vi "Untitled 1.vi"() -> ()   [LabVIEW 2010]
uses:
  Source Code/SubVIs/ModBUS Driver/Private/MBDRV_Action.ctl
  Source Code/SubVIs/ModBUS Driver/Private/MBDRV_Response.ctl
  Source Code/SubVIs/ModBUS Driver/Private/MBDRV_Response List.ctl
  Server/Serial Config.ctl
  Source Code/SubVIs/ModBUS Driver/Private/MBDRV_Command Data.ctl
  Source Code/SubVIs/ModBUS Driver/Private/MBDRV_Command List.ctl
  server.ctl
panel:
  in  "Radio Buttons":enum32{"Boolean", "Boolean 2", "Boolean 3"}(radio)
  in  "Tab Control":T1(tab)
  out "Response List":T2
  in  "Start":bool
  in  "Stop":bool
  in  "Exit":bool
  in  "Config":bool
  in  "Serial Config":T5={"串口选择"="COM1", "通讯速率"=9600, "超时时间"=200, "数据位长"=8, "奇偶校验"=enum."Even", "停止位长"=10, "握手控制"=0, "字符结束"=TRUE, "结束字符"=10, "仪器地址"=1, "刷新时间"=2.0} {"结束字符" format="%.0x"; "握手控制" items=["None", "XON/XOFF", "RTS/CTS", "XON/XOFF & RTS/CTS", "DTR/DSR", "XON/XOFF & DTR/DSR"]; "停止位长" items=["1.0"=10, "1.5"=15, "2.0"=20]; "数据位长" min=5 max=8 step=1}
  in  "Command":bool
  in  "Write To PLC":T6
  out "Read From PLC":T2
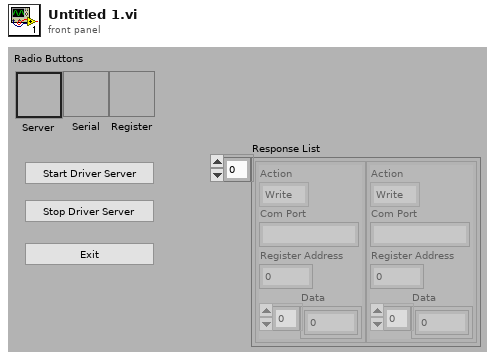
[diagram p1: front panel]
types:
  T1 = enum32{"Server Config", "Serial Config", "Write Registers"}
  T2 = typedef "MBDRV_Response List.ctl" = T3[]
  T3 = typedef "MBDRV_Response.ctl" = cluster{"Action":T4, "Com Port":string, "Register Address":u16, "Data":i16[]}
  T4 = typedef "MBDRV_Action.ctl" = enum16{"Write", "Read"}
  T5 = typedef "Serial Config.ctl" = cluster{"串口选择":refnum<visa-resource-name>, "通讯速率":u32, "超时时间":u32, "数据位长":u16, "奇偶校验":enum16{"None", "Odd", "Even", "Mark", "Space"}, "停止位长":u16, "握手控制":u16, "字符结束":bool, "结束字符":u8, "仪器地址":u32, "刷新时间":dbl}
  T6 = typedef "MBDRV_Command List.ctl" = T7[]
  T7 = typedef "MBDRV_Command Data.ctl" = cluster{"Action":T4, "Com Port":string, "Register Address":u16, "Data To Write/Num To Read":i16}
  T8 = typedef "LVRectTypeDef.ctl" = cluster{"left":i16, "top":i16, "right":i16, "bottom":i16}
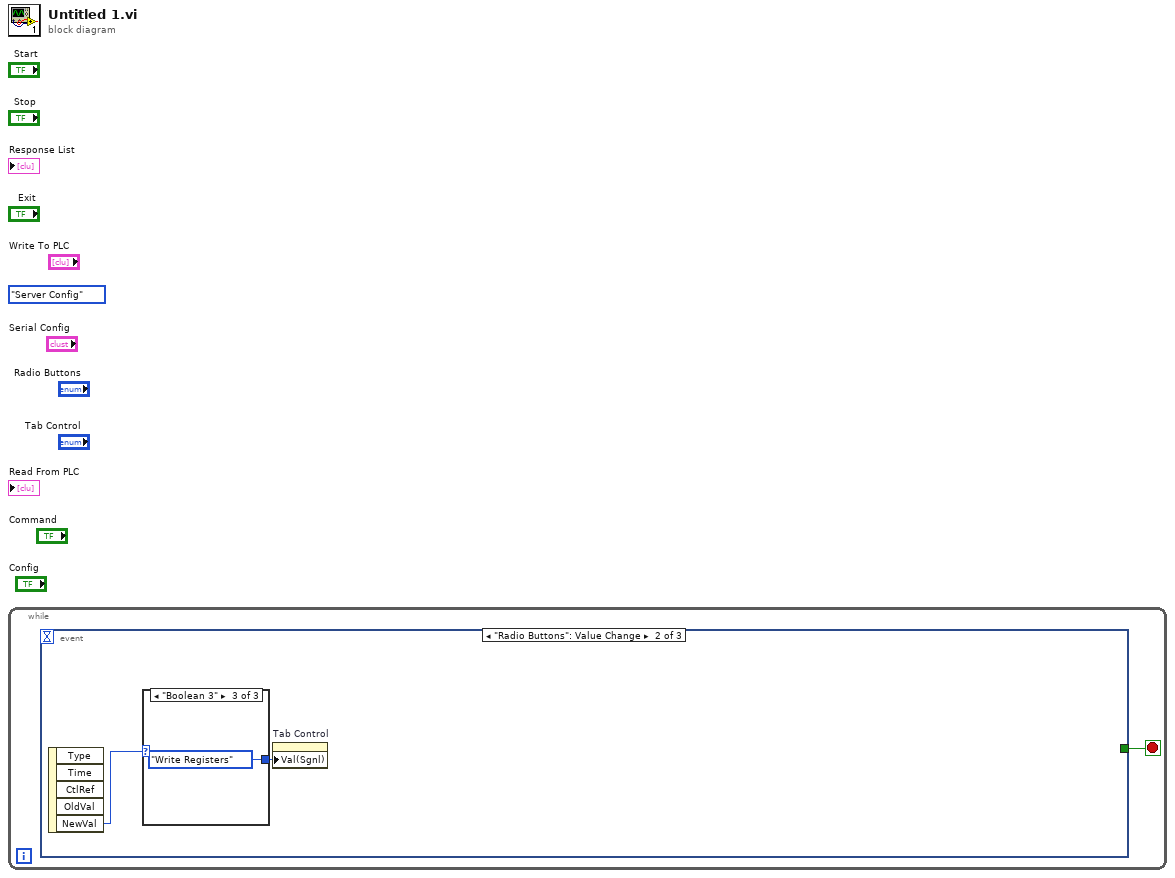
[diagram p0: block diagram]
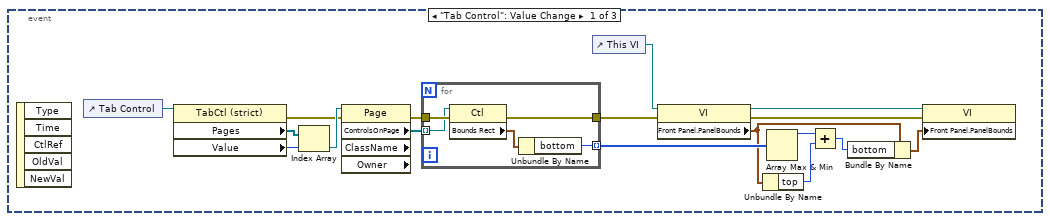
[diagram p2: hidden frame]
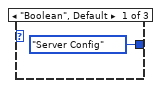
[diagram p3: hidden frame]
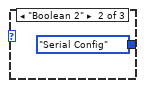
[diagram p4: hidden frame]
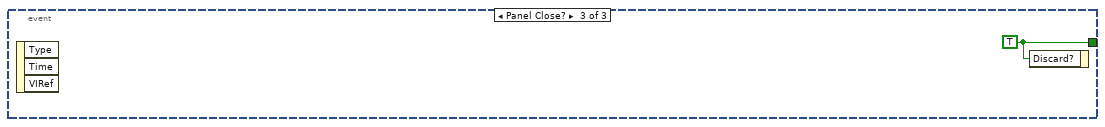
[diagram p5: hidden frame]
diagram:
  (unwired) T1."Server Config" ("Tab Control")
  n1 = while {
    stop <- w1 stop-if-true
    n2 = event shown="[1] \"Radio Buttons\": Value Change" {
      selector: _ -> [_ _ _]
      dyn-events: _ -> [_ _ _]
      timeout: _ -> [_ _ _]
      tunnel: [_ _ w29] -> w1
      event "Tab Control": Value Change {
        n3 = event-data() -> ()  [unwired: 1 in, 5 out]
        n4 = control-ref of="Tab Control"() -> (w4:refnum<vi>)
        n5 = property class="TabCtl (strict)"(reference=w4) -> (error out=w8:errorcluster, "Pages"=w18:refnum<vi>[], "Value"=w17:T1)  [unwired: 1 in, 1 out]
        n6 = Index Array(array=w18, index=w17) -> (element=w15:refnum<vi>)
        n7 = property class="Page" props=["ControlsOnPage", "ClassName", "Owner"](reference=w15, error in=w8) -> (error out=w7:errorcluster, "ControlsOnPage"=w16:refnum<vi>[])  [unwired: 3 out]
        n8 = for {
          tunnel: w16 -> [w19] mode=indexing
          tunnel: [w20] -> w14 mode=indexing
          tunnel: w7 -> [w23]
          tunnel: [w22] -> w6
          n9 = property class="Ctl"(reference=w19, error in=w23) -> (error out=w22:errorcluster, "Bounds Rect"=w21:T8)  [unwired: 1 out]
          n10 = Unbundle By Name(w21) -> ("bottom"=w20:i16)
        }
        n11 = control-ref of="This VI"() -> (w13:refnum<vi>)
        n12 = property class="VI"(reference=w13, error in=w6) -> (reference out=w12:refnum<vi>, error out=w5:errorcluster, "Front Panel.PanelBounds"=w3:T8)
        n13 = Unbundle By Name(w3) -> ("top"=w2:i16)
        n14 = Array Max & Min(array=w14) -> (max value=w11:i16)  [unwired: 3 out]
        n15 = Add(x=w11, y=w2) -> (x+y=w10:i16)
        n16 = Bundle By Name(cluster=w3, "bottom"=w10) -> (w9:T8)
        n17 = property class="VI"(reference=w12, error in=w5, "Front Panel.PanelBounds"=w9) -> ()  [unwired: 2 out]
      }
      event "Radio Buttons": Value Change {
        n18 = event-data() -> ("NewVal"=w24:enum32{"Boolean", "Boolean 2", "Boolean 3"})  [unwired: 1 in, 4 out]
        n19 = case shown="\"Boolean 3\"" w24 {
          tunnel: [T1."Server Config" ("Value (Signaling)") T1."Serial Config" ("Value (Signaling)") T1."Write Registers" ("Value (Signaling)")] -> w25
          frame "Boolean", Default {
          }
          frame "Boolean 2" {
          }
          frame "Boolean 3" {
          }
        }
        n20 = property on="Tab Control" class="TabCtl (strict)"("Val(Sgnl)"=w25) -> ()  [unwired: 2 in, 2 out]
      }
      event Panel Close? {
        w29 = TRUE ("Discard?")
        n21 = event-data() -> ()  [unwired: 1 in, 3 out]
        n22 = event-data("Discard?"=w29) -> ()  [unwired: 1 in, 1 out]
      }
    }
  }
